vi "Three part faster live.vi"() -> ()   [LabVIEW 2009]
uses:
  <vilib>/vision/Image Controls.llb/IMAQ Image.ctl
  <vilib>/Instr/_visa.llb/VISA Configure Serial Port (Instr).vi
  <vilib>/userDefined/High Color/IMAQdx.ctl
  <vilib>/Analysis/3filter.llb/Filter Passband Type.ctl
  <vilib>/Analysis/3filter.llb/Butterworth Filter (DBL).vi
  <vilib>/vision/NI_Vision_Development_Module.lvlib
  <vilib>/Analysis/NI_AALBase.lvlib
  <vilib>/vision/driver/NI_Vision_Acquisition_Software.lvlib
panel:
  out "Image 2":T1(plugin-control)
  out "decimal integer string 2":string
  out "number 2":u32
  out "cluster 2":T2
  in  "Orange Guitar":T3={"Global Rectangle"=[587, 282, 628, 378], "Contours"=[{"ID"=enum."External", "Type"=2, "Coordinates"=[627, 377, 587, 282]}]} {"Contours"."Type" items=["No Selection", "Point", "Line", "Rectangle", "Oval", "Polygon", "Freehand Region", "Annulus", "Unused2", "Unused3", "Broken Line", "Freehand Line", "Rotated Rectangle"]}
  in  "Yellow Guitar":T3={"Global Rectangle"=[546, 282, 563, 376], "Contours"=[{"ID"=enum."External", "Type"=2, "Coordinates"=[562, 375, 546, 282]}]} {"Contours"."Type" items=["No Selection", "Point", "Line", "Rectangle", "Oval", "Polygon", "Freehand Region", "Annulus", "Unused2", "Unused3", "Broken Line", "Freehand Line", "Rotated Rectangle"]}
  in  "Green Guitar":T3={"Global Rectangle"=[498, 284, 505, 376], "Contours"=[{"ID"=enum."External", "Type"=2, "Coordinates"=[498, 375, 504, 284]}]} {"Contours"."Type" items=["No Selection", "Point", "Line", "Rectangle", "Oval", "Polygon", "Freehand Region", "Annulus", "Unused2", "Unused3", "Broken Line", "Freehand Line", "Rotated Rectangle"]}
  in  "Blue Guitar":T3={"Global Rectangle"=[569, 290, 594, 372], "Contours"=[{"ID"=enum."External", "Type"=2, "Coordinates"=[593, 371, 569, 290]}]} {"Contours"."Type" items=["No Selection", "Point", "Line", "Rectangle", "Oval", "Polygon", "Freehand Region", "Annulus", "Unused2", "Unused3", "Broken Line", "Freehand Line", "Rotated Rectangle"]}
  in  "Red Guitar":T3={"Global Rectangle"=[526, 284, 530, 370], "Contours"=[{"ID"=enum."External", "Type"=2, "Coordinates"=[529, 369, 526, 284]}]} {"Contours"."Type" items=["No Selection", "Point", "Line", "Rectangle", "Oval", "Polygon", "Freehand Region", "Annulus", "Unused2", "Unused3", "Broken Line", "Freehand Line", "Rotated Rectangle"]}
  out "Blue Guitar":dbl[](graph)
  out "Yellow Guitar":dbl[](graph)
  out "Yellow Guitar LED":bool
  out "Green Guitar":dbl[](graph)
  out "Green Guitar LED":bool
  out "Red Guitar":dbl[](graph)
  out "Red Guitar LED":bool
  out "Blue Guitar LED":bool
  out "Orange Guitar":dbl[](graph)
  out "Orange Guitar LED":bool
  in  "Orange Bass":T3={"Global Rectangle"=[220, 296, 225, 371], "Contours"=[{"ID"=enum."External", "Type"=2, "Coordinates"=[224, 370, 220, 296]}]} {"Contours"."Type" items=["No Selection", "Point", "Line", "Rectangle", "Oval", "Polygon", "Freehand Region", "Annulus", "Unused2", "Unused3", "Broken Line", "Freehand Line", "Rotated Rectangle"]}
  out "Orange Bass":dbl[](graph)
  out "Orange Bass LED":bool
  in  "Green Bass":T3={"Global Rectangle"=[100, 292, 131, 371], "Contours"=[{"ID"=enum."External", "Type"=2, "Coordinates"=[100, 370, 130, 292]}]} {"Contours"."Type" items=["No Selection", "Point", "Line", "Rectangle", "Oval", "Polygon", "Freehand Region", "Annulus", "Unused2", "Unused3", "Broken Line", "Freehand Line", "Rotated Rectangle"]}
  in  "Blue Bass":T3={"Global Rectangle"=[193, 293, 199, 374], "Contours"=[{"ID"=enum."External", "Type"=2, "Coordinates"=[193, 373, 198, 293]}]} {"Contours"."Type" items=["No Selection", "Point", "Line", "Rectangle", "Oval", "Polygon", "Freehand Region", "Annulus", "Unused2", "Unused3", "Broken Line", "Freehand Line", "Rotated Rectangle"]}
  in  "Red Bass":T3={"Global Rectangle"=[129, 294, 154, 376], "Contours"=[{"ID"=enum."External", "Type"=2, "Coordinates"=[129, 375, 153, 294]}]} {"Contours"."Type" items=["No Selection", "Point", "Line", "Rectangle", "Oval", "Polygon", "Freehand Region", "Annulus", "Unused2", "Unused3", "Broken Line", "Freehand Line", "Rotated Rectangle"]}
  in  "Yellow Bass":T3={"Global Rectangle"=[160, 295, 175, 378], "Contours"=[{"ID"=enum."External", "Type"=2, "Coordinates"=[160, 377, 174, 295]}]} {"Contours"."Type" items=["No Selection", "Point", "Line", "Rectangle", "Oval", "Polygon", "Freehand Region", "Annulus", "Unused2", "Unused3", "Broken Line", "Freehand Line", "Rotated Rectangle"]}
  out "Blue Bass":dbl[](graph)
  out "Yellow Bass":dbl[](graph)
  out "Yellow Bass LED":bool
  out "Green Bass":dbl[](graph)
  out "Green Bass LED":bool
  out "Red Bass":dbl[](graph)
  out "Red Bass LED":bool
  out "Blue Bass LED":bool
  in  "Mask":T3 {"Contours"."Type" items=["No Selection", "Point", "Line", "Rectangle", "Oval", "Polygon", "Freehand Region", "Annulus", "Unused2", "Unused3", "Broken Line", "Freehand Line", "Rotated Rectangle"]}
  in  "Red Line":T3={"Global Rectangle"=[300, 297, 320, 380], "Contours"=[{"ID"=enum."External", "Type"=2, "Coordinates"=[300, 379, 319, 297]}]} {"Contours"."Type" items=["No Selection", "Point", "Line", "Rectangle", "Oval", "Polygon", "Freehand Region", "Annulus", "Unused2", "Unused3", "Broken Line", "Freehand Line", "Rotated Rectangle"]}
  out "Waveform Red":dbl[](graph)
  out "LED Red":bool
  in  "Blue Line":T3={"Global Rectangle"=[374, 278, 383, 377], "Contours"=[{"ID"=enum."External", "Type"=2, "Coordinates"=[382, 376, 374, 278]}]} {"Contours"."Type" items=["No Selection", "Point", "Line", "Rectangle", "Oval", "Polygon", "Freehand Region", "Annulus", "Unused2", "Unused3", "Broken Line", "Freehand Line", "Rotated Rectangle"]}
  in  "Green Line":T3={"Global Rectangle"=[406, 309, 423, 383], "Contours"=[{"ID"=enum."External", "Type"=2, "Coordinates"=[422, 382, 406, 309]}]} {"Contours"."Type" items=["No Selection", "Point", "Line", "Rectangle", "Oval", "Polygon", "Freehand Region", "Annulus", "Unused2", "Unused3", "Broken Line", "Freehand Line", "Rotated Rectangle"]}
  out "Waveform Green":dbl[](graph)
  out "LED Green":bool
  in  "Yellow Line":T3={"Global Rectangle"=[342, 292, 349, 377], "Contours"=[{"ID"=enum."External", "Type"=2, "Coordinates"=[342, 376, 348, 292]}]} {"Contours"."Type" items=["No Selection", "Point", "Line", "Rectangle", "Oval", "Polygon", "Freehand Region", "Annulus", "Unused2", "Unused3", "Broken Line", "Freehand Line", "Rotated Rectangle"]}
  out "cluster":T2
  in  "baud rate (9600)":u32=9600
  in  "VISA resource name":refnum<visa-resource-name>
  out "number":u32
  out "decimal integer string":string
  out "Image Dst Out":T1
  out "LED Yellow":bool
  out "Waveform Yellow":dbl[](graph)
  in  "playtime":dbl=30.0
  out "Frame Number":i32
  in  "Frame Start":i32=2400
  out "Blue Drum":bool
  out "Blue Drum":dbl[](graph)
  in  "stop":bool
  # "Drums"
  # "Bass"
  # "Guitar"
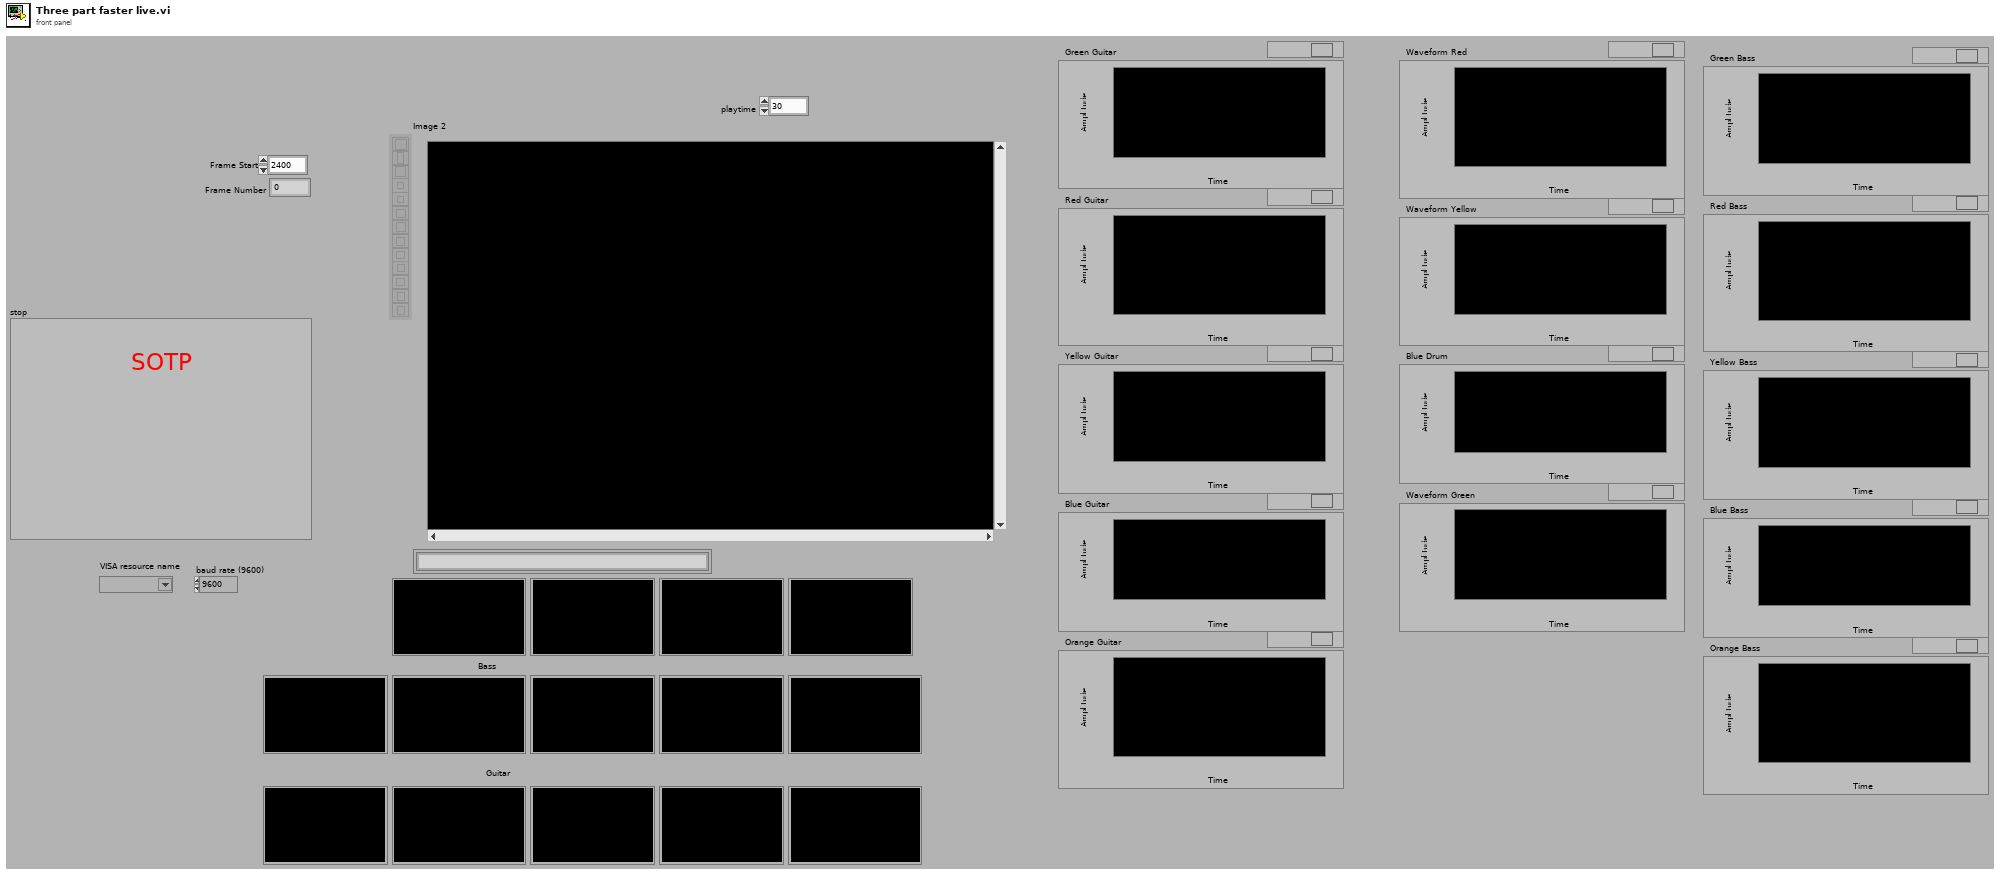
[diagram p1: front panel]
types:
  T1 = typedef "IMAQ Image.ctl" = refnum<image>
  T2 = cluster{"[0]":bool, "[1]":bool, "[2]":bool, "[3]":bool, "[4]":bool, "[5]":bool, "[6]":bool, "[7]":bool, "[8]":bool}
  T3 = cluster{"Global Rectangle":i32[], "Contours":cluster{"ID":enum32{"External", "Internal"}, "Type":u32, "Coordinates":i32[]}[]}
  T4 = typedef "IMAQdx.ctl" = refnum<k21>
  T5 = typedef "NI_AALBase.lvlib/Filter Passband Type.ctl" = enum32{"Lowpass", "Highpass", "Bandpass", "Bandstop"}
  T6 = typedef "Image Type" = u32
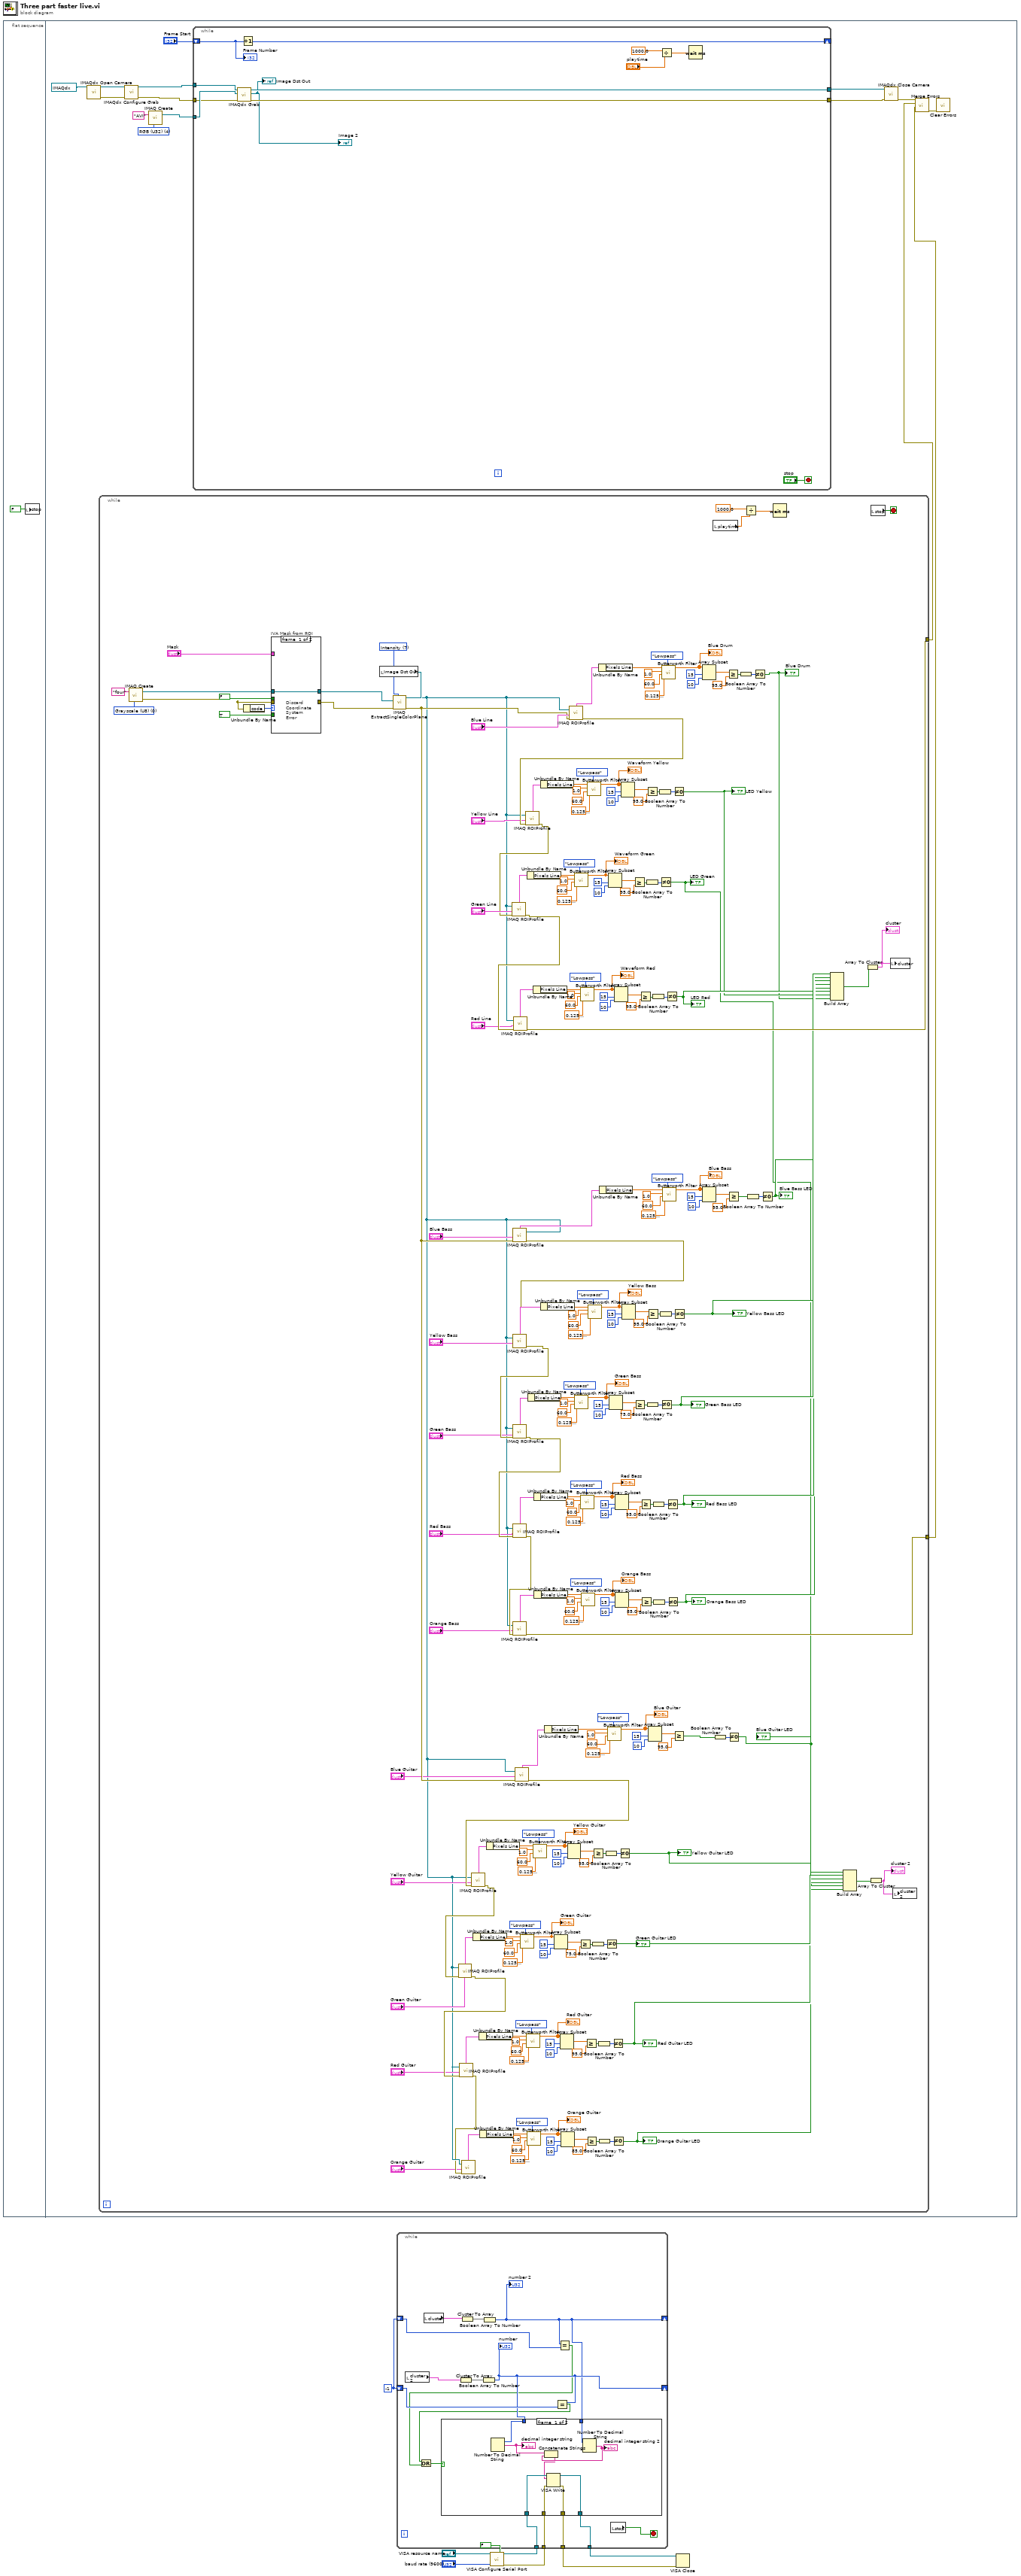
[diagram p0: block diagram]
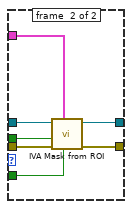
[diagram p3: hidden frame]
diagram:
  w1 = -1
  n1 = flat-sequence {
    frame #0 {
      n2 = local write "stop"(FALSE ("stop")) -> ()
    }
    frame #1 {
      w20 = T6 4 items=["Grayscale (U8)", "Grayscale (I16)", "Grayscale (SGL)", "Complex (CSG)", "RGB (U32)", "HSL (U32)", "RGB (U64)", "Grayscale (U16)"] ("Image Type")
      n3 = call <vilib>:"IMAQdx Open Camera.vi"("Session In"=T4 "cam0") -> ("error out"=w18:errorcluster, "Session Out"=w17:T4)  [unwired: 9 in]
      n4 = while {
        tunnel: [w253] -> w22
        tunnel: [w119] -> w21
        stop <- w268 stop-if-true
        w263 = T6 0 items=["Grayscale (U8)", "Grayscale (I16)", "Grayscale (SGL)", "Complex (CSG)", "RGB (U32)", "HSL (U32)", "RGB (U64)", "Grayscale (U16)"] ("Image Type")
        w269 = 7 items=["Red", "Green", "Blue", "Hue", "Saturation", "Luminance", "Value", "Intensity"] ("Color Plane")
        n5 = call "IMAQ Create"("Image Name"="four", "Image Type"=w263) -> ("New Image"=w256:T1, "error out"=w257:errorcluster)  [unwired: 3 in]
        n6 = Unbundle By Name(w257) -> ("code"=w261:i32)
        n7 = case "IVA Mask from ROI" shown="Default" w261 {
          tunnel: "Mask" -> [_ w277]
          tunnel: TRUE ("Shrink") -> [_ w276]
          tunnel: w256 -> [w270 w275]
          tunnel: w257 -> [_ w274]
          tunnel: [_ w273] -> w258
          tunnel: [w270 w272] -> w254
          tunnel: FALSE ("Out / In") -> [_ w271]
          frame #0 {
            # "Discard\nCoordinate\nSystem\nError"
          }
          frame #1 {
            n8 = call <vilib>:"IVA Mask from ROI.vi"("Shrink"=w276, "ROI Descriptor"=w277, "error in (no error)"=w274, "Out / In"=w271, "Image Src"=w275) -> ("error out"=w273:errorcluster, "Image Out"=w272:T1)  [unwired: 5 out]
          }
        }
        n9 = local read "Image Dst Out"() -> (w264:T1)
        n10 = call "IMAQ ExtractSingleColorPlane"("Color Plane"=w269, "error in (no error)"=w258, "Image Dst"=w254, "Image Src"=w264) -> ("error out"=w41:errorcluster, "Image Dst Out"=w36:T1)  [unwired: 6 out]
        n11 = call "IMAQ ROIProfile"("error in (no error)"=w41, "ROI Descriptor"="Blue Bass", "Image"=w36) -> ("error out"=w168:errorcluster, "ROI Graph"=w167:cluster{"x0":sgl, "dx":sgl, "Pixels Line":sgl[]})  [unwired: 4 out]
        n12 = call "IMAQ ROIProfile"("error in (no error)"=w168, "ROI Descriptor"="Yellow Bass", "Image"=w36) -> ("error out"=w138:errorcluster, "ROI Graph"=w171:cluster{"x0":sgl, "dx":sgl, "Pixels Line":sgl[]})  [unwired: 4 out]
        n13 = call "IMAQ ROIProfile"("error in (no error)"=w138, "ROI Descriptor"="Green Bass", "Image"=w36) -> ("error out"=w139:errorcluster, "ROI Graph"=w165:cluster{"x0":sgl, "dx":sgl, "Pixels Line":sgl[]})  [unwired: 4 out]
        n14 = call "IMAQ ROIProfile"("error in (no error)"=w139, "ROI Descriptor"="Red Bass", "Image"=w36) -> ("error out"=w120:errorcluster, "ROI Graph"=w141:cluster{"x0":sgl, "dx":sgl, "Pixels Line":sgl[]})  [unwired: 4 out]
        n15 = call "IMAQ ROIProfile"("error in (no error)"=w120, "ROI Descriptor"="Orange Bass", "Image"=w36) -> ("error out"=w119:errorcluster, "ROI Graph"=w132:cluster{"x0":sgl, "dx":sgl, "Pixels Line":sgl[]})  [unwired: 4 out]
        n16 = call "IMAQ ROIProfile"("error in (no error)"=w41, "ROI Descriptor"="Blue Guitar", "Image"=w36) -> ("error out"=w65:errorcluster, "ROI Graph"=w66:cluster{"x0":sgl, "dx":sgl, "Pixels Line":sgl[]})  [unwired: 4 out]
        n17 = call "IMAQ ROIProfile"("error in (no error)"=w65, "ROI Descriptor"="Yellow Guitar", "Image"=w36) -> ("error out"=w95:errorcluster, "ROI Graph"=w62:cluster{"x0":sgl, "dx":sgl, "Pixels Line":sgl[]})  [unwired: 4 out]
        n18 = call "IMAQ ROIProfile"("error in (no error)"=w95, "ROI Descriptor"="Green Guitar", "Image"=w36) -> ("error out"=w94:errorcluster, "ROI Graph"=w68:cluster{"x0":sgl, "dx":sgl, "Pixels Line":sgl[]})  [unwired: 4 out]
        n19 = call "IMAQ ROIProfile"("error in (no error)"=w94, "ROI Descriptor"="Red Guitar", "Image"=w36) -> ("error out"=w35:errorcluster, "ROI Graph"=w92:cluster{"x0":sgl, "dx":sgl, "Pixels Line":sgl[]})  [unwired: 4 out]
        n20 = call "IMAQ ROIProfile"("error in (no error)"=w35, "ROI Descriptor"="Orange Guitar", "Image"=w36) -> ("ROI Graph"=w34:cluster{"x0":sgl, "dx":sgl, "Pixels Line":sgl[]})  [unwired: 5 out]
        n21 = Unbundle By Name(w68) -> ("Pixels Line"=w71:sgl[])
        n22 = Unbundle By Name(w92) -> ("Pixels Line"=w89:sgl[])
        n23 = Unbundle By Name(w34) -> ("Pixels Line"=w99:sgl[])
        n24 = Unbundle By Name(w62) -> ("Pixels Line"=w59:sgl[])
        n25 = call-poly <vilib>:"Butterworth Filter.vi"("filter type"=Filter_Passband_Type."Lowpass", "low cutoff freq: fl"=0.12500000000000006 ("low  11"), "high cutoff freq: fh"=60.0 ("high 12"), "sampling freq: fs"=1.0 ("sampling 11"), "X"=w71) -> ("Filtered X"=w67:dbl[])  [unwired: 3 in, 1 out]
        "Green Guitar" <- w67
        n26 = call-poly <vilib>:"Butterworth Filter.vi"("filter type"=Filter_Passband_Type."Lowpass", "low cutoff freq: fl"=0.12500000000000006 ("low  10"), "high cutoff freq: fh"=60.0 ("high 11"), "sampling freq: fs"=1.0 ("sampling 10"), "X"=w89) -> ("Filtered X"=w93:dbl[])  [unwired: 3 in, 1 out]
        "Red Guitar" <- w93
        n27 = call-poly <vilib>:"Butterworth Filter.vi"("filter type"=Filter_Passband_Type."Lowpass", "low cutoff freq: fl"=0.12500000000000006 ("low  9"), "high cutoff freq: fh"=60.0 ("high 10"), "sampling freq: fs"=1.0 ("sampling 9"), "X"=w99) -> ("Filtered X"=w96:dbl[])  [unwired: 3 in, 1 out]
        "Orange Guitar" <- w96
        n28 = Unbundle By Name(w165) -> ("Pixels Line"=w162:sgl[])
        n29 = call-poly <vilib>:"Butterworth Filter.vi"("filter type"=Filter_Passband_Type."Lowpass", "low cutoff freq: fl"=0.12500000000000006 ("low  12"), "high cutoff freq: fh"=60.0 ("high 13"), "sampling freq: fs"=1.0 ("sampling 12"), "X"=w59) -> ("Filtered X"=w63:dbl[])  [unwired: 3 in, 1 out]
        "Yellow Guitar" <- w63
        n30 = Unbundle By Name(w141) -> ("Pixels Line"=w144:sgl[])
        n31 = Unbundle By Name(w132) -> ("Pixels Line"=w129:sgl[])
        n32 = Unbundle By Name(w171) -> ("Pixels Line"=w174:sgl[])
        n33 = Unbundle By Name(w66) -> ("Pixels Line"=w43:sgl[])
        n34 = Array Subset(array=w67, index=15, length=10) -> (w76:dbl[])
        n35 = Array Subset(array=w93, index=15, length=10) -> (w84:dbl[])
        n36 = Array Subset(array=w96, index=15, length=10) -> (w104:dbl[])
        n37 = Array Subset(array=w63, index=15, length=10) -> (w54:dbl[])
        n38 = call "IMAQ ROIProfile"("error in (no error)"=w41, "ROI Descriptor"="Blue Line", "Image"=w36) -> ("error out"=w228:errorcluster, "ROI Graph"=w227:cluster{"x0":sgl, "dx":sgl, "Pixels Line":sgl[]})  [unwired: 4 out]
        n39 = call "IMAQ ROIProfile"("error in (no error)"=w228, "ROI Descriptor"="Yellow Line", "Image"=w36) -> ("error out"=w195:errorcluster, "ROI Graph"=w231:cluster{"x0":sgl, "dx":sgl, "Pixels Line":sgl[]})  [unwired: 4 out]
        n40 = call "IMAQ ROIProfile"("error in (no error)"=w195, "ROI Descriptor"="Green Line", "Image"=w36) -> ("error out"=w198:errorcluster, "ROI Graph"=w225:cluster{"x0":sgl, "dx":sgl, "Pixels Line":sgl[]})  [unwired: 4 out]
        n41 = call "IMAQ ROIProfile"("error in (no error)"=w198, "ROI Descriptor"="Red Line", "Image"=w36) -> ("error out"=w253:errorcluster, "ROI Graph"=w200:cluster{"x0":sgl, "dx":sgl, "Pixels Line":sgl[]})  [unwired: 4 out]
        n42 = Unbundle By Name(w225) -> ("Pixels Line"=w222:sgl[])
        n43 = Unbundle By Name(w200) -> ("Pixels Line"=w203:sgl[])
        n44 = Unbundle By Name(w231) -> ("Pixels Line"=w234:sgl[])
        n45 = call-poly <vilib>:"Butterworth Filter.vi"("filter type"=Filter_Passband_Type."Lowpass", "low cutoff freq: fl"=0.12500000000000006 ("low  3"), "high cutoff freq: fh"=60.0 ("high 3"), "sampling freq: fs"=1.0 ("sampling 3"), "X"=w222) -> ("Filtered X"=w226:dbl[])  [unwired: 3 in, 1 out]
        "Waveform Green" <- w226
        n46 = call-poly <vilib>:"Butterworth Filter.vi"("filter type"=Filter_Passband_Type."Lowpass", "low cutoff freq: fl"=0.12500000000000006 ("low  6"), "high cutoff freq: fh"=60.0 ("high 6"), "sampling freq: fs"=1.0 ("sampling 6"), "X"=w162) -> ("Filtered X"=w166:dbl[])  [unwired: 3 in, 1 out]
        "Green Bass" <- w166
        n47 = Greater Or Equal?(x=w76, y=75.0) -> (x >= y?=w74:bool[])
        n48 = call-poly <vilib>:"Butterworth Filter.vi"("filter type"=Filter_Passband_Type."Lowpass", "low cutoff freq: fl"=0.12500000000000006 ("low  4"), "high cutoff freq: fh"=60.0 ("high 4"), "sampling freq: fs"=1.0 ("sampling 4"), "X"=w203) -> ("Filtered X"=w199:dbl[])  [unwired: 3 in, 1 out]
        "Waveform Red" <- w199
        n49 = call-poly <vilib>:"Butterworth Filter.vi"("filter type"=Filter_Passband_Type."Lowpass", "low cutoff freq: fl"=0.12500000000000006 ("low  5"), "high cutoff freq: fh"=60.0 ("high 5"), "sampling freq: fs"=1.0 ("sampling 5"), "X"=w144) -> ("Filtered X"=w140:dbl[])  [unwired: 3 in, 1 out]
        "Red Bass" <- w140
        n50 = call-poly <vilib>:"Butterworth Filter.vi"("filter type"=Filter_Passband_Type."Lowpass", "low cutoff freq: fl"=0.12500000000000006 ("low  8"), "high cutoff freq: fh"=60.0 ("high 9"), "sampling freq: fs"=1.0 ("sampling 8"), "X"=w129) -> ("Filtered X"=w133:dbl[])  [unwired: 3 in, 1 out]
        "Orange Bass" <- w133
        n51 = Greater Or Equal?(x=w84, y=95.0) -> (x >= y?=w86:bool[])
        n52 = Greater Or Equal?(x=w104, y=85.0) -> (x >= y?=w102:bool[])
        n53 = call-poly <vilib>:"Butterworth Filter.vi"("filter type"=Filter_Passband_Type."Lowpass", "low cutoff freq: fl"=0.12500000000000006 ("low  2"), "high cutoff freq: fh"=60.0 ("high 2"), "sampling freq: fs"=1.0 ("sampling 2"), "X"=w234) -> ("Filtered X"=w230:dbl[])  [unwired: 3 in, 1 out]
        "Waveform Yellow" <- w230
        n54 = call-poly <vilib>:"Butterworth Filter.vi"("filter type"=Filter_Passband_Type."Lowpass", "low cutoff freq: fl"=0.12500000000000006 ("low  7"), "high cutoff freq: fh"=60.0 ("high 7"), "sampling freq: fs"=1.0 ("sampling 7"), "X"=w174) -> ("Filtered X"=w170:dbl[])  [unwired: 3 in, 1 out]
        "Yellow Bass" <- w170
        n55 = Boolean Array To Number(Boolean array=w74) -> (number=w73:u32)
        n56 = Greater Or Equal?(x=w54, y=95.0) -> (x >= y?=w56:bool[])
        n57 = Boolean Array To Number(Boolean array=w86) -> (number=w87:u32)
        n58 = Boolean Array To Number(Boolean array=w102) -> (number=w101:u32)
        n59 = Unbundle By Name(w227) -> ("Pixels Line"=w251:sgl[])
        n60 = Unbundle By Name(w167) -> ("Pixels Line"=w190:sgl[])
        n61 = Boolean Array To Number(Boolean array=w56) -> (number=w57:u32)
        n62 = Not Equal To 0?(x=w73) -> (x != 0?=w31:bool)
        "Green Guitar LED" <- w31
        n63 = call-poly <vilib>:"Butterworth Filter.vi"("filter type"=Filter_Passband_Type."Lowpass", "low cutoff freq: fl"=0.12500000000000006 ("low 3"), "high cutoff freq: fh"=60.0 ("high 14"), "sampling freq: fs"=1.0 ("sampling  9"), "X"=w43) -> ("Filtered X"=w80:dbl[])  [unwired: 3 in, 1 out]
        "Blue Guitar" <- w80
        n64 = Array Subset(array=w226, index=15, length=10) -> (w217:dbl[])
        n65 = Array Subset(array=w166, index=15, length=10) -> (w157:dbl[])
        n66 = Not Equal To 0?(x=w87) -> (x != 0?=w30:bool)
        "Red Guitar LED" <- w30
        n67 = Not Equal To 0?(x=w101) -> (x != 0?=w27:bool)
        "Orange Guitar LED" <- w27
        n68 = Array Subset(array=w199, index=15, length=10) -> (w208:dbl[])
        n69 = Array Subset(array=w140, index=15, length=10) -> (w149:dbl[])
        n70 = Array Subset(array=w133, index=15, length=10) -> (w124:dbl[])
        n71 = Not Equal To 0?(x=w57) -> (x != 0?=w29:bool)
        "Yellow Guitar LED" <- w29
        n72 = Array Subset(array=w230, index=15, length=10) -> (w239:dbl[])
        n73 = Array Subset(array=w170, index=15, length=10) -> (w179:dbl[])
        n74 = Greater Or Equal?(x=w217, y=95.0) -> (x >= y?=w219:bool[])
        n75 = Greater Or Equal?(x=w157, y=75.0) -> (x >= y?=w159:bool[])
        n76 = Greater Or Equal?(x=w208, y=95.0) -> (x >= y?=w206:bool[])
        n77 = Greater Or Equal?(x=w149, y=95.0) -> (x >= y?=w147:bool[])
        n78 = Greater Or Equal?(x=w124, y=85.0) -> (x >= y?=w126:bool[])
        n79 = Boolean Array To Number(Boolean array=w219) -> (number=w220:u32)
        n80 = Greater Or Equal?(x=w239, y=95.0) -> (x >= y?=w237:bool[])
        n81 = Boolean Array To Number(Boolean array=w159) -> (number=w160:u32)
        n82 = Greater Or Equal?(x=w179, y=95.0) -> (x >= y?=w177:bool[])
        n83 = Array Subset(array=w80, index=15, length=10) -> (w49:dbl[])
        n84 = Boolean Array To Number(Boolean array=w206) -> (number=w205:u32)
        n85 = Boolean Array To Number(Boolean array=w147) -> (number=w146:u32)
        n86 = Boolean Array To Number(Boolean array=w126) -> (number=w127:u32)
        n87 = Boolean Array To Number(Boolean array=w237) -> (number=w236:u32)
        n88 = Boolean Array To Number(Boolean array=w177) -> (number=w176:u32)
        n89 = Not Equal To 0?(x=w220) -> (x != 0?=w32:bool)
        "LED Green" <- w32
        n90 = Not Equal To 0?(x=w160) -> (x != 0?=w117:bool)
        "Green Bass LED" <- w117
        n91 = call-poly <vilib>:"Butterworth Filter.vi"("filter type"=Filter_Passband_Type."Lowpass", "low cutoff freq: fl"=0.12500000000000006 ("low"), "high cutoff freq: fh"=60.0 ("high"), "sampling freq: fs"=1.0 ("sampling"), "X"=w251) -> ("Filtered X"=w213:dbl[])  [unwired: 3 in, 1 out]
        "Blue Drum" <- w213
        n92 = call-poly <vilib>:"Butterworth Filter.vi"("filter type"=Filter_Passband_Type."Lowpass", "low cutoff freq: fl"=0.12500000000000006 ("low 2"), "high cutoff freq: fh"=60.0 ("high 8"), "sampling freq: fs"=1.0 ("sampling  8"), "X"=w190) -> ("Filtered X"=w153:dbl[])  [unwired: 3 in, 1 out]
        "Blue Bass" <- w153
        n93 = Not Equal To 0?(x=w205) -> (x != 0?=w112:bool)
        "LED Red" <- w112
        n94 = Not Equal To 0?(x=w146) -> (x != 0?=w116:bool)
        "Red Bass LED" <- w116
        n95 = Not Equal To 0?(x=w127) -> (x != 0?=w113:bool)
        "Orange Bass LED" <- w113
        n96 = Not Equal To 0?(x=w236) -> (x != 0?=w111:bool)
        "LED Yellow" <- w111
        n97 = Greater Or Equal?(x=w49, y=95.0) -> (x >= y?=w108:bool[])
        n98 = Not Equal To 0?(x=w176) -> (x != 0?=w115:bool)
        "Yellow Bass LED" <- w115
        n99 = Array Subset(array=w213, index=15, length=10) -> (w245:dbl[])
        n100 = Array Subset(array=w153, index=15, length=10) -> (w184:dbl[])
        n101 = local read "playtime"() -> (w265:dbl)
        n102 = Boolean Array To Number(Boolean array=w108) -> (number=w51:u32)
        n103 = Greater Or Equal?(x=w245, y=95.0) -> (x >= y?=w243:bool[])
        n104 = Greater Or Equal?(x=w184, y=95.0) -> (x >= y?=w109:bool[])
        n105 = Not Equal To 0?(x=w51) -> (x != 0?=w28:bool)
        "Blue Guitar LED" <- w28
        n106 = Boolean Array To Number(Boolean array=w243) -> (number=w242:u32)
        n107 = Divide(x=1000.0, y=w265) -> (x/y=w267:dbl)
        n108 = Boolean Array To Number(Boolean array=w109) -> (number=w182:u32)
        n109 = Not Equal To 0?(x=w242) -> (x != 0?=w110:bool)
        "Blue Drum" <- w110
        n110 = Not Equal To 0?(x=w182) -> (x != 0?=w114:bool)
        "Blue Bass LED" <- w114
        n111 = Wait (ms)(milliseconds to wait=w267) -> ()  [unwired: 1 out]
        n112 = Build Array(w117, w116, w115, w114, w113, w112, w111, w110) -> (w193:bool[])
        n113 = Build Array(w32, w31, w30, w29, w28, w27) -> (w26:bool[])
        n114 = Array To Cluster(array=w193) -> (cluster=w194:T2)
        "cluster" <- w194
        n115 = Array To Cluster(array=w26) -> (cluster=w25:T2)
        "cluster 2" <- w25
        n116 = local read "stop"() -> (w268:bool)
        n117 = local write "cluster"(w194) -> ()
        n118 = local write "cluster 2"(w25) -> ()
      }
      n119 = call <vilib>:"IMAQdx Configure Grab.vi"("error in"=w18, "Session In"=w17) -> ("error out"=w15:errorcluster, "Session Out"=w14:T4)  [unwired: 8 in]
      n120 = call "IMAQ Create"("Image Name"="AVI", "Image Type"=w20) -> ("New Image"=w13:T1)  [unwired: 3 in, 1 out]
      n121 = while {
        tunnel: [w279] -> w10
        shift-right: [w285] -> _
        shift-left: "Frame Start" -> [w284]
        tunnel: [w280] -> w12
        tunnel: w13 -> [w283]
        tunnel: w15 -> [w282]
        tunnel: w14 -> [w281]
        stop <- "stop" stop-if-true
        n122 = call <vilib>:"IMAQdx Grab.vi"("error in"=w282, "Image In"=w283, "Session In"=w281) -> ("error out"=w280:errorcluster, "Image Out"=→"Image Dst Out" →"Image 2":T1, "Session Out"=w279:T4)  [unwired: 5 in, 1 out]
        n123 = Increment(x=w284) -> (x+1=w285:i32)
        n124 = Divide(x=1000.0, y="playtime") -> (x/y=w288:dbl)
        n125 = Wait (ms)(milliseconds to wait=w288) -> ()  [unwired: 1 out]
        "Frame Number" <- w284
      }
      n126 = call <vilib>:"IMAQdx Close Camera.vi"("error in"=w12, "Session In"=w10) -> ("error out"=w11:errorcluster)  [unwired: 9 in]
      n127 = call <vilib>:"Merge Errors.vi"("error in 3 (no error)"=w21, "error in 2 (no error)"=w22, "error in 1 (no error)"=w11) -> ("error out"=w23:errorcluster)  [unwired: 4 in]
      n128 = call <vilib>:"Clear Errors.vi"("error in (no error)"=w23) -> ()  [unwired: 6 in, 1 out]
    }
  }
  n129 = call-poly "VISA Configure Serial Port"("VISA resource name"="VISA resource name", "Enable Termination\nChar (T)"=FALSE ("Enable Termination\nChar (T)"), "baud rate (9600)"="baud rate (9600)") -> ("VISA resource name out"=w8:refnum<visa-resource-name>, "error out"=w3:errorcluster)  [unwired: 11 in]
  n130 = while {
    shift-right: [w294] -> _
    shift-left: w1 -> [w305]
    tunnel: w8 -> [w304]
    tunnel: [w303] -> w7
    tunnel: w3 -> [w302]
    tunnel: [w301] -> w2
    shift-right: [w293] -> _
    shift-left: w1 -> [w297]
    stop <- w299 stop-if-true
    n131 = local read "cluster 2"() -> (w295:T2)
    n132 = local read "cluster"() -> (w296:T2)
    n133 = Cluster To Array(cluster=w295) -> (array=w300:bool[])
    n134 = Cluster To Array(cluster=w296) -> (array=w298:bool[])
    n135 = Boolean Array To Number(Boolean array=w300) -> (number=w294:u32)
    "number" <- w294
    n136 = Boolean Array To Number(Boolean array=w298) -> (number=w293:u32)
    "number 2" <- w293
    n137 = Equal?(x=w294, y=w305) -> (x = y?=w292:bool)
    n138 = Equal?(x=w293, y=w297) -> (x = y?=w291:bool)
    n139 = Or(x=w292, y=w291) -> (x .or. y?=w290:bool)
    n140 = case shown="False" w290 {
      tunnel: w304 -> [w314 w316]
      tunnel: [w313 w316] -> w303
      tunnel: w294 -> [w312 _]
      tunnel: w302 -> [w311 w315]
      tunnel: [w310 w315] -> w301
      tunnel: w293 -> [w309 _]
      frame #0 {
        n141 = Number To Decimal String(number=w312) -> (decimal integer string=w308:string)  [unwired: 1 in]
        "decimal integer string" <- w308
        n142 = Number To Decimal String(number=w309) -> (decimal integer string=w307:string)  [unwired: 1 in]
        "decimal integer string 2" <- w307
        n143 = Concatenate Strings(w308, w307) -> (w306:string)
        n144 = VISA Write(VISA resource name=w314, write buffer=w306, error in (no error)=w311) -> (VISA resource name out=w313:refnum<visa-resource-name>, error out=w310:errorcluster)  [unwired: 1 out]
      }
      frame #1 {
      }
    }
    n145 = local read "stop"() -> (w299:bool)
  }
  n146 = VISA Close(VISA resource name=w7, error in (no error)=w2) -> ()  [unwired: 1 out]
